vi "TD_PKYK_User.vi"() -> (3 "User":string)   [LabVIEW 2020]
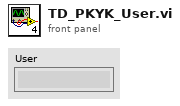
[diagram p1: front panel]
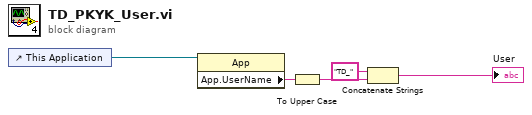
[diagram p0: block diagram]
diagram:
  n1 = control-ref of="This Application"() -> (w1:refnum<vi>)
  n2 = property class="App"(reference=w1) -> ("App.UserName"=w2:string)  [unwired: 1 in, 2 out]
  n3 = To Upper Case(1:w2) -> (0:w3:string)
  n4 = Concatenate Strings("TD_" ("string"), w3) -> (→"User":string)
